vi "Init_can.vi"(8 "entrée d'erreur (pas d'erreur)":errorcluster, 11 "X-CAN en entrée":refnum<class "X-CAN.lvclass">) -> (0 "sortie d'erreur":errorcluster, 3 "X-CAN en sortie":refnum<class "X-CAN.lvclass">)   [LabVIEW 2014]
uses:
  <vilib>/Stratom, Inc/X-CAN for myRIO (API)/X-CAN Class/X-CAN.lvclass
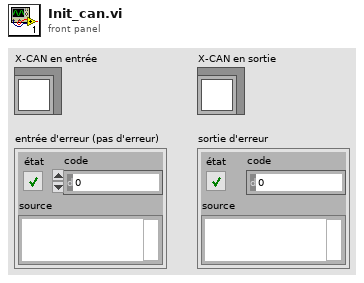
[diagram p1: front panel]
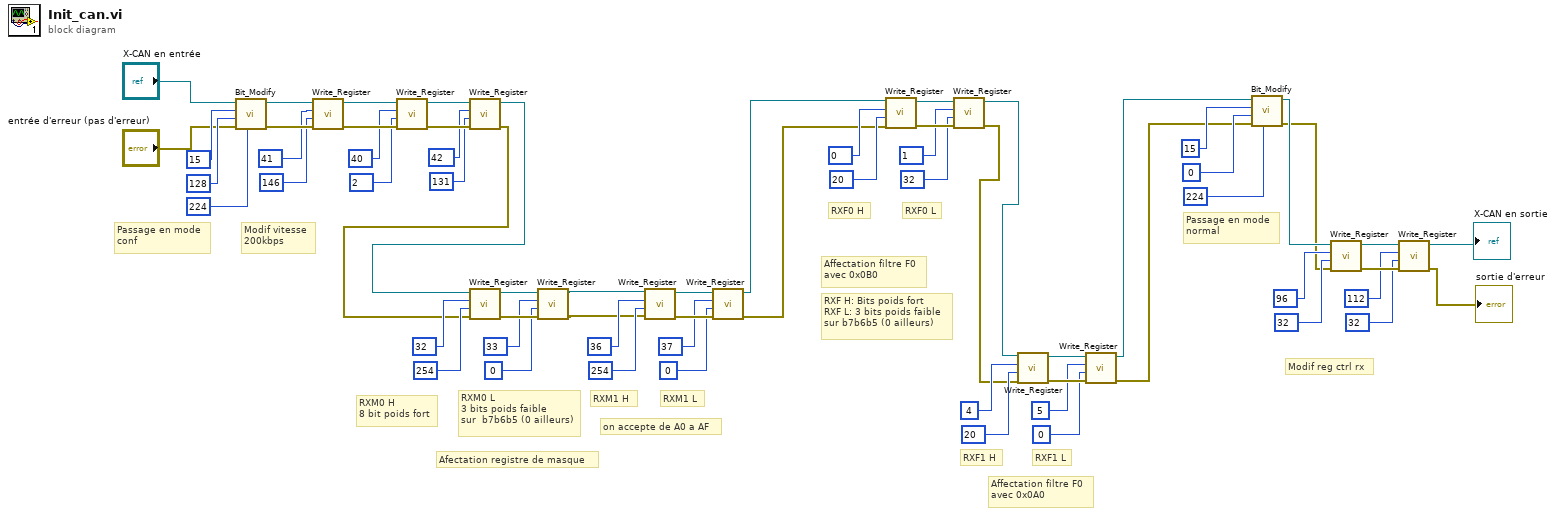
[diagram p0: block diagram]
diagram:
  # "on accepte de A0 a AF"
  # "RXF1 L"
  # "RXF1 H"
  # "RXF0 L"
  # "RXF0 H"
  # "RXF H: Bits poids fort\nRXF L: 3 bits poids faible\nsur b7b6b5 (0 ailleurs)"
  # "RXM1 L"
  # "RXM1 H"
  # "RXM0 L\n3 bits poids faible\nsur  b7b6b5 (0 ailleurs)"
  # "RXM0 H\n8 bit poids fort"
  # "Affectation filtre F0\navec 0x0A0"
  # "Affectation filtre F0\navec 0x0B0"
  # "Afectation registre de masque"
  # "Modif reg ctrl rx"
  # "Passage en mode\nnormal"
  # "Modif vitesse\n200kbps"
  # "Passage en mode\nconf"
  n1 = call <vilib>:"Bit_Modify.vi"("Mask Byte"=u8 224, "error in"="entrée d'erreur (pas d'erreur)", "Write Byte"=u8 128, "Register"=u8 15, "X-CAN Session in"="X-CAN en entrée") -> ("error out"=w58:errorcluster, "X-CAN Session out"=w56:refnum<class "X-CAN.lvclass">)  [unwired: 5 in]
  n2 = call <vilib>:"Write_Register.vi"("error in"=w58, "Write Byte"=u8 146, "Register"=u8 41, "X-CAN Session in"=w56) -> ("error out"=w9:errorcluster, "X-CAN Session out"=w10:refnum<class "X-CAN.lvclass">)  [unwired: 6 in]
  n3 = call <vilib>:"Write_Register.vi"("error in"=w9, "Write Byte"=u8 2, "Register"=u8 40, "X-CAN Session in"=w10) -> ("error out"=w7:errorcluster, "X-CAN Session out"=w8:refnum<class "X-CAN.lvclass">)  [unwired: 6 in]
  n4 = call <vilib>:"Write_Register.vi"("error in"=w7, "Write Byte"=u8 131, "Register"=u8 42, "X-CAN Session in"=w8) -> ("error out"=w6:errorcluster, "X-CAN Session out"=w5:refnum<class "X-CAN.lvclass">)  [unwired: 6 in]
  n5 = call <vilib>:"Write_Register.vi"("error in"=w6, "Write Byte"=u8 254, "Register"=u8 32, "X-CAN Session in"=w5) -> ("error out"=w46:errorcluster, "X-CAN Session out"=w45:refnum<class "X-CAN.lvclass">)  [unwired: 6 in]
  n6 = call <vilib>:"Write_Register.vi"("error in"=w46, "Write Byte"=u8 0, "Register"=u8 33, "X-CAN Session in"=w45) -> ("error out"=w33:errorcluster, "X-CAN Session out"=w34:refnum<class "X-CAN.lvclass">)  [unwired: 6 in]
  n7 = call <vilib>:"Write_Register.vi"("error in"=w33, "Write Byte"=u8 254, "Register"=u8 36, "X-CAN Session in"=w34) -> ("error out"=w40:errorcluster, "X-CAN Session out"=w39:refnum<class "X-CAN.lvclass">)  [unwired: 6 in]
  n8 = call <vilib>:"Write_Register.vi"("error in"=w40, "Write Byte"=u8 0, "Register"=u8 37, "X-CAN Session in"=w39) -> ("error out"=w25:errorcluster, "X-CAN Session out"=w26:refnum<class "X-CAN.lvclass">)  [unwired: 6 in]
  n9 = call <vilib>:"Write_Register.vi"("error in"=w25, "Write Byte"=u8 20, "Register"=u8 0, "X-CAN Session in"=w26) -> ("error out"=w32:errorcluster, "X-CAN Session out"=w31:refnum<class "X-CAN.lvclass">)  [unwired: 6 in]
  n10 = call <vilib>:"Write_Register.vi"("error in"=w32, "Write Byte"=u8 32, "Register"=u8 1, "X-CAN Session in"=w31) -> ("error out"=w13:errorcluster, "X-CAN Session out"=w14:refnum<class "X-CAN.lvclass">)  [unwired: 6 in]
  n11 = call <vilib>:"Write_Register.vi"("error in"=w13, "Write Byte"=u8 20, "Register"=u8 4, "X-CAN Session in"=w14) -> ("error out"=w20:errorcluster, "X-CAN Session out"=w19:refnum<class "X-CAN.lvclass">)  [unwired: 6 in]
  n12 = call <vilib>:"Write_Register.vi"("error in"=w20, "Write Byte"=u8 0, "Register"=u8 5, "X-CAN Session in"=w19) -> ("error out"=w11:errorcluster, "X-CAN Session out"=w12:refnum<class "X-CAN.lvclass">)  [unwired: 6 in]
  n13 = call <vilib>:"Bit_Modify.vi"("Mask Byte"=u8 224, "error in"=w11, "Write Byte"=u8 0, "Register"=u8 15, "X-CAN Session in"=w12) -> ("error out"=w23:errorcluster, "X-CAN Session out"=w24:refnum<class "X-CAN.lvclass">)  [unwired: 5 in]
  n14 = call <vilib>:"Write_Register.vi"("error in"=w23, "Write Byte"=u8 32, "Register"=u8 96, "X-CAN Session in"=w24) -> ("error out"=w52:errorcluster, "X-CAN Session out"=w51:refnum<class "X-CAN.lvclass">)  [unwired: 6 in]
  n15 = call <vilib>:"Write_Register.vi"("error in"=w52, "Write Byte"=u8 32, "Register"=u8 112, "X-CAN Session in"=w51) -> ("error out"=→"sortie d'erreur":errorcluster, "X-CAN Session out"=→"X-CAN en sortie":refnum<class "X-CAN.lvclass">)  [unwired: 6 in]
